vi "Destroy.vi"(8 "error in (no error)":errorcluster, 11 "ConfigManagerCollection in":refnum<class "ConfigManagerCollection.lvclass">) -> (0 "error out":errorcluster, 3 "ConfigManagerCollection out":refnum<class "ConfigManagerCollection.lvclass">)   [LabVIEW 2013, in "CfgManager.lvlib" / "ConfigManagerCollection.lvclass"]
uses:
  ConfigManagerCollection.lvclass
  Manager/ConfigManager.lvclass
  ConfigManagerCollection.lvclass/ConfigManagerCollection.ctl
  Cache/ConfigManager.Cache.lvclass
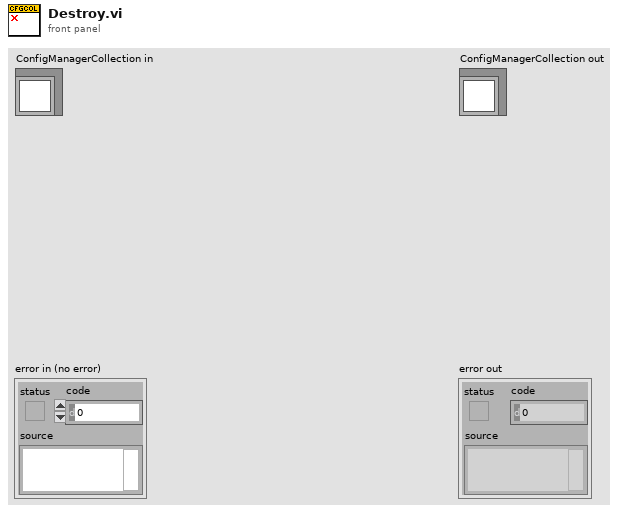
[diagram p1: front panel]
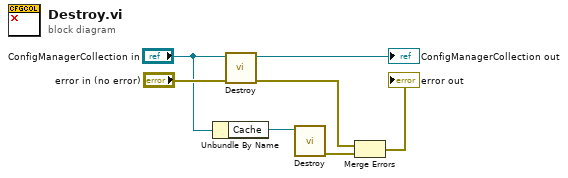
[diagram p0: block diagram]
diagram:
  n1 = Unbundle By Name("ConfigManagerCollection in") -> ("Cache"=w4:refnum<class "ConfigManager.Cache.lvclass">)
  n2 = call-parent "Destroy.vi"("error in (no error)"="error in (no error)", "ConfigManager in"="ConfigManagerCollection in") -> ("error out"=w2:errorcluster, "ConfigManager out"=→"ConfigManagerCollection out":refnum<class "ConfigManagerCollection.lvclass">)  [unwired: 8 in]
  n3 = call-dynamic "Destroy.vi"("ConfigManager.Cache in"=w4) -> ("error out"=w3:errorcluster)  [unwired: 9 in, 1 out]
  n4 = Merge Errors(w2, w3) -> (→"error out":errorcluster)
